vi "InitializeAndor.vi"(3 "Error In":errorcluster) -> (0 "error out":errorcluster, 1 "Andor Initialization Error Codes":T2, 2 "Camera Information":T1 {"VS Speed (us)" format="%.2f"})   [LabVIEW 2013]
uses:
  states.ctl
  CameraTest/System Files/user.lib/atmcd32d.llb/Error Code Enum typedef.ctl
panel:
  in  "Camera Inputs":cluster{"Path":path}
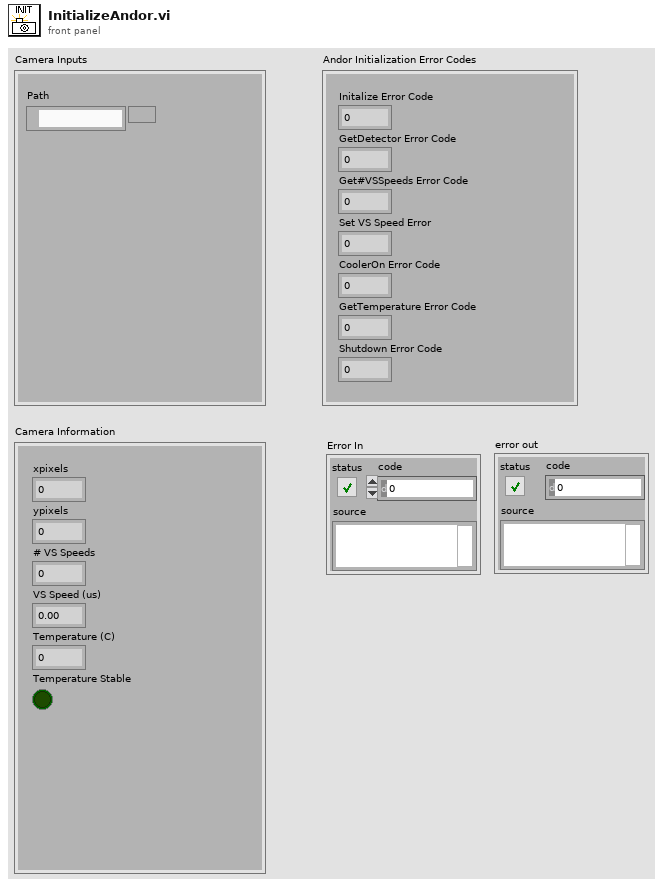
[diagram p1: front panel]
types:
  T1 = cluster{"xpixels":i32, "ypixels":i32, "# VS Speeds":i32, "VS Speed (us)":sgl, "Temperature Stable":bool, "Temperature (C)":i32}
  T2 = cluster{"Initalize Error Code":u32, "GetDetector Error Code":u32, "Get#VSSpeeds Error Code":u32, "Set VS Speed Error":u32, "CoolerOn Error Code":u32, "GetTemperature Error Code":u32, "Shutdown Error Code":u32}
  T3 = typedef "states.ctl" = enum16{"Initialize", "Turn on Cooler", "Close With No Error", "Shutdown"}
  T4 = typedef "Error Code Enum typedef.ctl" = enum32{"N/A (0)", "DRV_ERROR_CODES", "DRV_SUCCESS", "DRV_VXDNOTINSTALLED", "DRV_ERROR_SCAN", "DRV_ERROR_CHECK_SUM", "DRV_ERROR_FILELOAD", "DRV_UNKNOWN_FUNC", "DRV_ERROR_VXD_INIT", "DRV_ERROR_ADDRESS", "DRV_ERROR_PAGELOCK", "DRV_ERROR_PAGEUNLOCK", "DRV_ERROR_BOARDTEST", "DRV_ERROR_ACK", "DRV_ERROR_UP_FIFO", "DRV_ERROR_PATTERN", "N/A (16)", "DRV_ACQUISITION_ERRORS", "DRV_ACQ_BUFFER", "DRV_ACQ_DOWNFIFO_FULL", "DRV_PROC_UNKONWN_INSTRUCTION", "DRV_ILLEGAL_OP_CODE", "DRV_KINETIC_TIME_NOT_MET", "DRV_ACCUM_TIME_NOT_MET", "DRV_NO_NEW_DATA", "N/A (25)", "DRV_SPOOLERROR", "N/A (27)", "N/A (28)", "N/A (29)", "N/A (30)", "N/A (31)", "N/A (32)", "DRV_TEMPERATURE_CODES", "DRV_TEMPERATURE_OFF", "DRV_TEMPERATURE_NOT_STABILIZED", "DRV_TEMPERATURE_STABILIZED", "DRV_TEMPERATURE_NOT_REACHED", "DRV_TEMPERATURE_OUT_RANGE", "DRV_TEMPERATURE_NOT_SUPPORTED", "DRV_TEMPERATURE_DRIFT", "N/A (41)", "N/A (42)", "N/A (43)", "N/A (44)", "N/A (45)", "N/A (46)", "N/A (47)", "N/A (48)", "DRV_GENERAL_ERRORS", "DRV_INVALID_AUX", "DRV_COF_NOTLOADED", "DRV_FPGAPROG", "DRV_FLEXERROR", "DRV_GPIBERROR", "N/A (55)", "N/A (56)", "N/A (57)", "N/A (58)", "N/A (59)", "N/A (60)", "N/A (61)", "N/A (62)", "N/A (63)", "DRV_DATATYPE", "DRV_DRIVER_ERRORS", "DRV_P1INVALID", "DRV_P2INVALID", "DRV_P3INVALID", "DRV_P4INVALID", "DRV_INIERROR", "DRV_COFERROR", "DRV_ACQUIRING", "DRV_IDLE", "DRV_TEMPCYCLE", "DRV_NOT_INITIALIZED", "DRV_P5INVALID", "DRV_P6INVALID", "DRV_INVALID_MODE", "DRV_INVALID_FILTER", "DRV_I2CERRORS", "DRV_I2CDEVNOTFOUND", "DRV_I2CTIMEOUT", "DRV_P7INVALID", "N/A (84)", "N/A (85)", "N/A (86)", "N/A (87)", "N/A (88)", "N/A (89)", "DRV_IOCERROR", "DRV_VRMVERSIONERROR"}
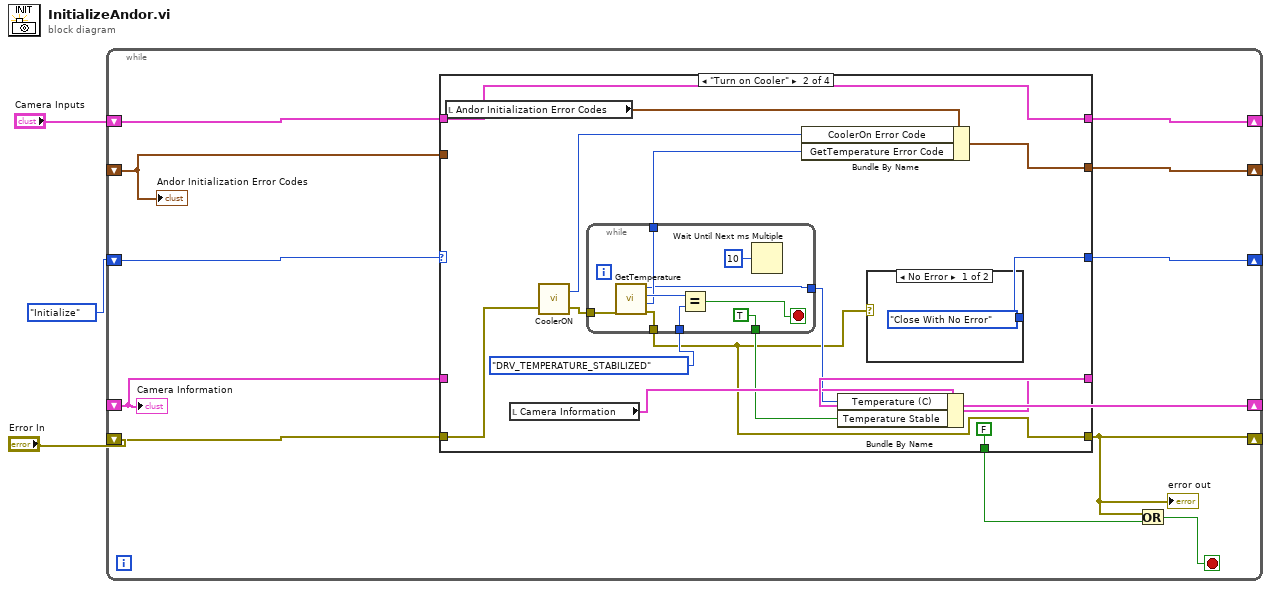
[diagram p0: block diagram]
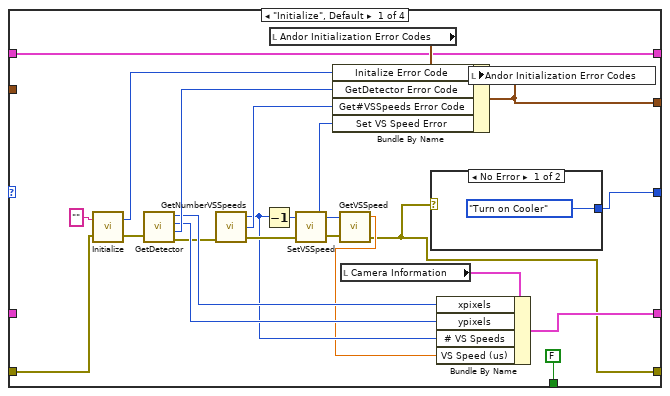
[diagram p2: hidden frame]
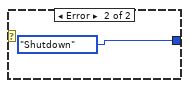
[diagram p3: hidden frame]
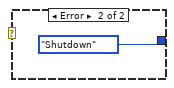
[diagram p4: hidden frame]
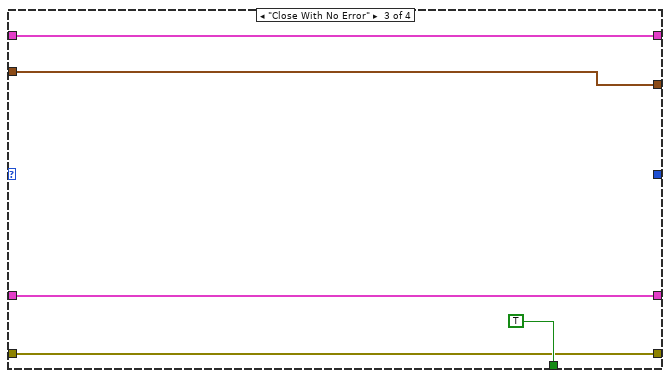
[diagram p5: hidden frame]
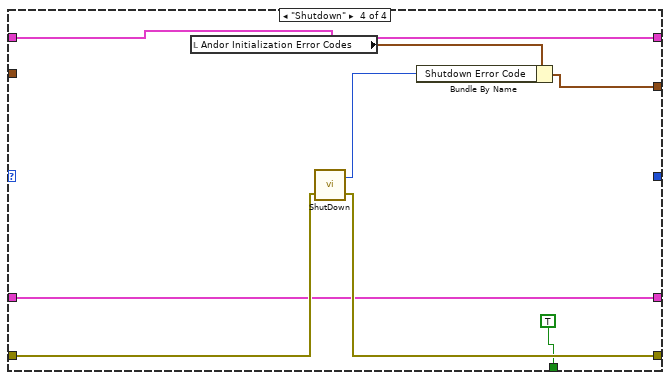
[diagram p6: hidden frame]
diagram:
  n1 = while {
    shift-right: [w11] -> _
    shift-left: states."Initialize" -> [w15]
    shift-right: [w6] -> _
    shift-left: "Error In" -> [w7]
    shift-right: [w14] -> _
    shift-left: _ -> [w4]
    shift-right: [w13] -> _
    shift-left: "Camera Inputs" -> [w12]
    shift-right: [w8] -> _
    shift-left: _ -> [w5]
    stop <- w9 stop-if-true
    n2 = case shown="\"Turn on Cooler\"" w15 {
      tunnel: [w16 w43 w69 w78] -> w6
      tunnel: w7 -> [w37 w54 w69 w79]
      tunnel: [w32 w51 w67 w75] -> w14
      tunnel: [FALSE FALSE TRUE TRUE] -> w10
      tunnel: [w33 w41 w70 w74] -> w13
      tunnel: w12 -> [w33 w41 w70 w74]
      tunnel: [w17 w42 _ _] -> w11
      tunnel: [w24 w44 w68 w72] -> w8
      tunnel: w5 -> [_ _ w68 w72]
      tunnel: w4 -> [_ _ w67 _]
      frame "Initialize", Default {
        n3 = call <userlib>:"Initialize.vi"("error in (no error)"=w37, "directory (\"\")"="" ("directory (\"\")")) -> ("error out"=w31:errorcluster, "DLL error code"=w35:u32)
        n4 = call <userlib>:"GetDetector.vi"("error in (no error)"=w31) -> ("error out"=w26:errorcluster, "DLL error code"=w30:u32, "ypixels"=w27:i32, "xpixels"=w28:i32)  [unwired: 3 in]
        n5 = call <userlib>:"GetNumberVSSpeeds.vi"("error in (no error)"=w26) -> ("error out"=w23:errorcluster, "DLL error code"=w25:u32, "number"=w22:i32)  [unwired: 2 in]
        n6 = Decrement(x=w22) -> (x-1=w19:i32)
        n7 = local read "Andor Initialization Error Codes"() -> (w36:T2)
        n8 = call <userlib>:"SetVSSpeed.vi"("error in (no error)"=w23, "index"=w19) -> ("error out"=w20:errorcluster, "DLL error code"=w21:u32)
        n9 = Bundle By Name(cluster=w36, "Initalize Error Code"=w35, "GetDetector Error Code"=w30, "Get#VSSpeeds Error Code"=w25, "Set VS Speed Error"=w21) -> (w32:T2)
        n10 = call <userlib>:"GetVSSpeed.vi"("error in (no error)"=w20, "index"=w19) -> ("error out"=w16:errorcluster, "speed"=w18:sgl)  [unwired: 1 in, 1 out]
        n11 = local read "Camera Information"() -> (w29:T1)
        n12 = case shown="No Error" w16 {
          tunnel: [states."Turn on Cooler" states."Shutdown"] -> w17
          frame No Error {
          }
          frame Error {
          }
        }
        n13 = Bundle By Name(cluster=w29, "xpixels"=w28, "ypixels"=w27, "# VS Speeds"=w22, "VS Speed (us)"=w18) -> (w24:T1)
        n14 = local write "Andor Initialization Error Codes"(w32) -> ()
      }
      frame "Turn on Cooler" {
        n15 = local read "Andor Initialization Error Codes"() -> (w53:T2)
        n16 = local read "Camera Information"() -> (w47:T1)
        n17 = call <userlib>:"CoolerON.vi"("error in (no error)"=w54) -> ("error out"=w50:errorcluster, "DLL error code"=w52:u32)  [unwired: 1 in]
        n18 = while {
          tunnel: w50 -> [w66]
          tunnel: Error_Code_Enum_typedef."DRV_TEMPERATURE_STABILIZED" ("y") -> [w64]
          tunnel: [w63] -> w48
          tunnel: [w62] -> w46
          tunnel: [TRUE] -> w45
          tunnel: [w58] -> w43
          stop <- w61 stop-if-true
          n19 = call <userlib>:"GetTemperature.vi"("error in (no error)"=w66) -> ("error out"=w58:errorcluster, "DLL error code"=w63:u32, "status"=w65:T4, "temperature"=w62:i32)  [unwired: 3 in]
          n20 = Equal?(x=w65, y=w64) -> (x = y?=w61:bool)
          n21 = Wait Until Next ms Multiple(millisecond multiple=u32 10) -> ()  [unwired: 1 out]
        }
        n22 = Bundle By Name(cluster=w53, "CoolerOn Error Code"=w52, "GetTemperature Error Code"=w48) -> (w51:T2)
        n23 = Bundle By Name(cluster=w47, "Temperature (C)"=w46, "Temperature Stable"=w45) -> (w44:T1)
        n24 = case shown="No Error" w43 {
          tunnel: [states."Close With No Error" states."Shutdown"] -> w42
          frame No Error {
          }
          frame Error {
          }
        }
      }
      frame "Close With No Error" {
      }
      frame "Shutdown" {
        n25 = local read "Andor Initialization Error Codes"() -> (w77:T2)
        n26 = call <userlib>:"ShutDown.vi"("error in (no error)"=w79) -> ("error out"=w78:errorcluster, "DLL error code"=w76:u32)  [unwired: 1 in]
        n27 = Bundle By Name(cluster=w77, "Shutdown Error Code"=w76) -> (w75:T2)
      }
    }
    "error out" <- w6
    n28 = Or(x=w6, y=w10) -> (x .or. y?=w9:bool)
    "Andor Initialization Error Codes" <- w4
    "Camera Information" <- w5
  }
